vi "BottleLayerGen.vi"(6 "Layer":u32=160, 10 "HatchPow":T6={"Power"=300.0, "Mark Speed"=400.0, "Jump Speed"=1000.0}, 11 "CircHatch":T1={"Diameter"=1.0, "Angle"=45.0, "Offset"=0.1, "Spacing"=0.1} {"Spacing" format="%#_13g"; "Offset" format="%#_13g"; "Diameter" format="%#_13g"}) -> (3 "PathSups":T2[](array[typedef]))   [LabVIEW 2014]
uses:
  TypeDefs/PowerSpeed.ctl
  TypeDefs/PathSupreme.ctl
  PSup2SCAN/Sub/VelocityProfile.ctl
  PSup2SCAN/Sub/PathCut.ctl
  PSup2SCAN/Sub/Segment.ctl
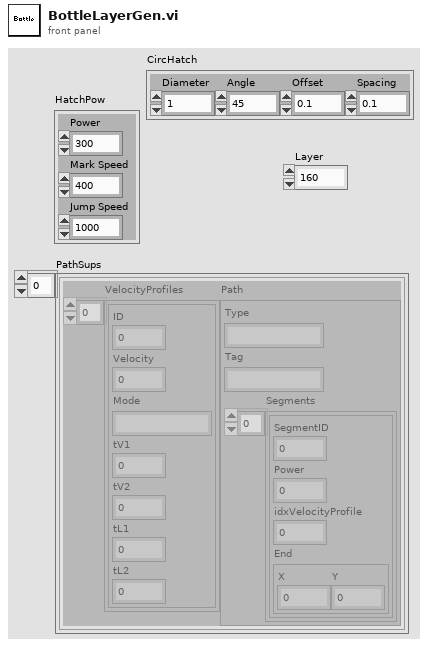
[diagram p1: front panel]
types:
  T1 = cluster{"Diameter":dbl, "Angle":sgl, "Offset":dbl, "Spacing":dbl}
  T2 = typedef "PathSupreme.ctl" = cluster{"VelocityProfiles":T3[], "Path":T4}
  T3 = typedef "VelocityProfile.ctl" = cluster{"ID":u32, "Velocity":dbl, "Mode":string, "tV1":u32, "tV2":u32, "tL1":u32, "tL2":u32}
  T4 = typedef "PathCut.ctl" = cluster{"Type":string, "Tag":string, "Segments":T5[]}
  T5 = typedef "Segment.ctl" = cluster{"SegmentID":u16, "Power":sgl, "idxVelocityProfile":u16, "End":cluster{"X":sgl, "Y":sgl}}
  T6 = typedef "PowerSpeed.ctl" = cluster{"Power":dbl, "Mark Speed":dbl, "Jump Speed":dbl}
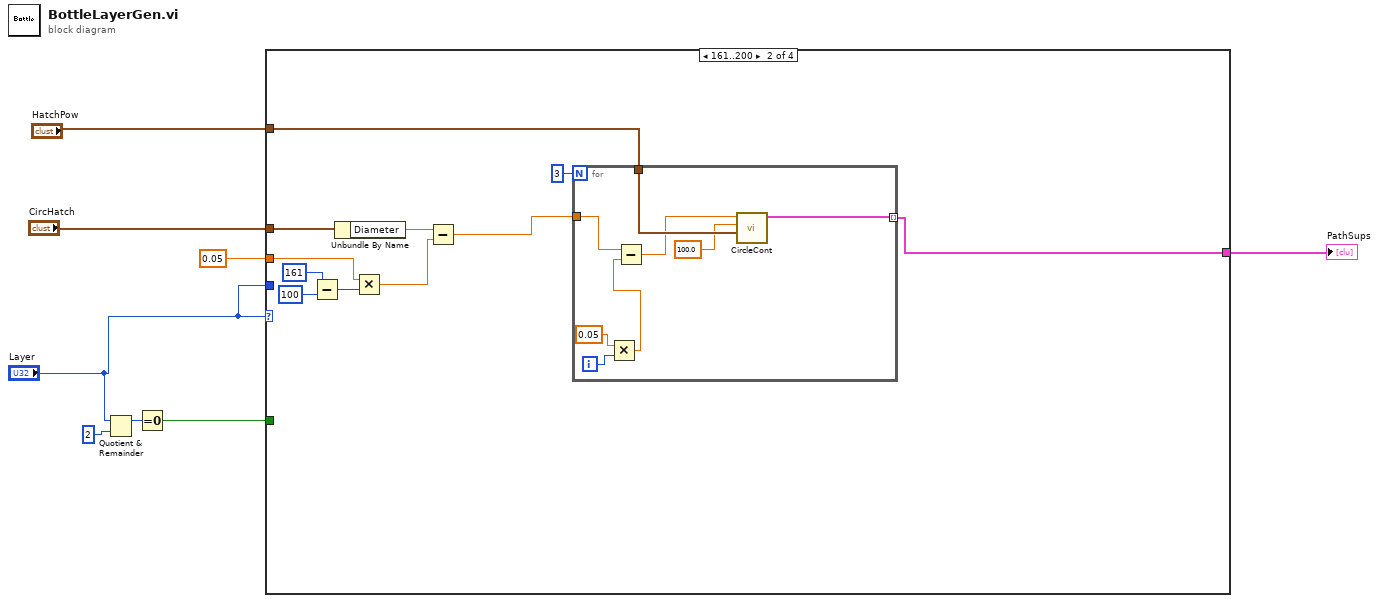
[diagram p0: block diagram]
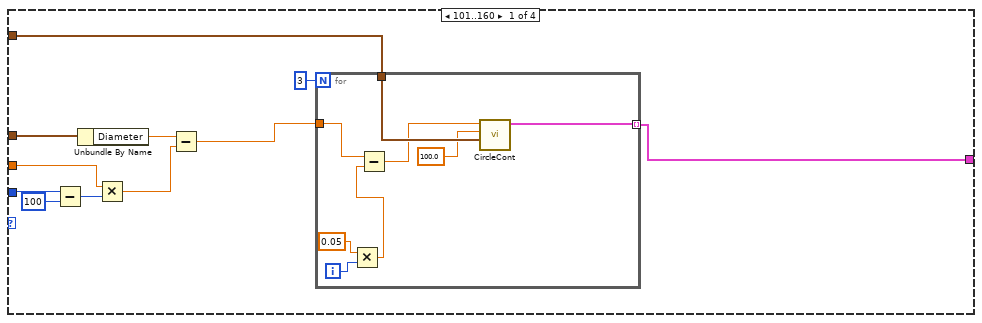
[diagram p2: hidden frame]
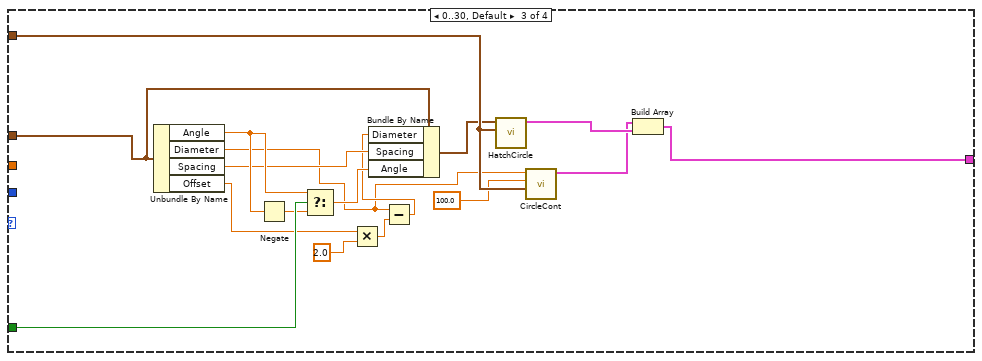
[diagram p3: hidden frame]
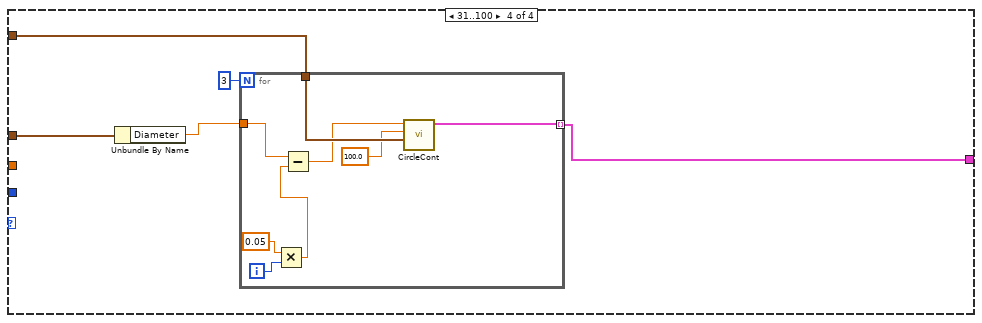
[diagram p4: hidden frame]
diagram:
  n1 = Quotient & Remainder(x="Layer", y=u8 2) -> (x-y*floor(x/y)=w8:u32)  [unwired: 1 out]
  n2 = Equal To 0?(x=w8) -> (x = 0?=w6:bool)
  n3 = case shown="161..200" "Layer" {
    tunnel: w6 -> [_ _ w63 _]
    tunnel: "HatchPow" -> [w18 w37 w62 w68]
    tunnel: [w9 w28 w61 w64] -> w4
    tunnel: "CircHatch" -> [w17 w36 w54 w67]
    tunnel: "Layer" -> [w15 _ _ _]
    tunnel: 0.05 -> [w11 w31 _ _]
    frame 101..160 {
      n4 = Subtract(x=w15, y=u32 100) -> (x-y=w13:u32)
      n5 = Unbundle By Name(w17) -> ("Diameter"=w16:dbl)
      n6 = Multiply(x=w11, y=w13) -> (x*y=w12:dbl)
      n7 = Subtract(x=w16, y=w12) -> (x-y=w10:dbl)
      n8 = for {
        N: 3 -> [_]
        tunnel: w18 -> [w27]
        tunnel: w10 -> [w25]
        tunnel: [w20] -> w9 mode=indexing
        i -> [w24]
        n9 = Multiply(x=0.05, y=w24) -> (x*y=w22:dbl)
        n10 = Subtract(x=w25, y=w22) -> (x-y=w21:dbl)
        n11 = call "CircleCont.vi"("ContPow"=w27, "NumSides"=100.0, "Diameter"=w21) -> ("PathSupreme"=w20:T2)  [unwired: 8 in]
      }
    }
    frame 161..200 {
      n12 = Subtract(x=u32 161, y=u32 100) -> (x-y=w33:u32)
      n13 = Unbundle By Name(w36) -> ("Diameter"=w35:dbl)
      n14 = Multiply(x=w31, y=w33) -> (x*y=w32:dbl)
      n15 = Subtract(x=w35, y=w32) -> (x-y=w30:dbl)
      n16 = for {
        N: 3 -> [_]
        tunnel: w37 -> [w46]
        tunnel: w30 -> [w44]
        tunnel: [w39] -> w28 mode=indexing
        i -> [w43]
        n17 = Multiply(x=0.05, y=w43) -> (x*y=w41:dbl)
        n18 = Subtract(x=w44, y=w41) -> (x-y=w40:dbl)
        n19 = call "CircleCont.vi"("ContPow"=w46, "NumSides"=100.0, "Diameter"=w40) -> ("PathSupreme"=w39:T2)  [unwired: 8 in]
      }
    }
    frame 0..30, Default {
      n20 = Unbundle By Name(w54) -> ("Angle"=w59:sgl, "Diameter"=w47:dbl, "Spacing"=w56:dbl, "Offset"=w52:dbl)
      n21 = Negate(x=w59) -> (-x=w60:sgl)
      n22 = Select(t=w59, s=w63, f=w60) -> (s? t:f=w58:sgl)
      n23 = Multiply(x=w52, y=2.0) -> (x*y=w51:dbl)
      n24 = Subtract(x=w47, y=w51) -> (x-y=w48:dbl)
      n25 = Bundle By Name(cluster=w54, "Diameter"=w48, "Spacing"=w56, "Angle"=w58) -> (w57:T1)
      n26 = call "HatchCircle.vi"("HatchPow"=w62, "CircHatch"=w57) -> ("PathSupreme"=w55:T2)  [unwired: 9 in]
      n27 = call "CircleCont.vi"("ContPow"=w62, "NumSides"=100.0, "Diameter"=w47) -> ("PathSupreme"=w49:T2)  [unwired: 8 in]
      n28 = Build Array(w49, w55) -> (w61:T2[])
    }
    frame 31..100 {
      n29 = Unbundle By Name(w67) -> ("Diameter"=w66:dbl)
      n30 = for {
        N: 3 -> [_]
        tunnel: w68 -> [w76]
        tunnel: w66 -> [w74]
        tunnel: [w69] -> w64 mode=indexing
        i -> [w73]
        n31 = Multiply(x=0.05, y=w73) -> (x*y=w71:dbl)
        n32 = Subtract(x=w74, y=w71) -> (x-y=w70:dbl)
        n33 = call "CircleCont.vi"("ContPow"=w76, "NumSides"=100.0, "Diameter"=w70) -> ("PathSupreme"=w69:T2)  [unwired: 8 in]
      }
    }
  }
  "PathSups" <- w4
